vi "Connect CAN Adapter.vi"(8 "error in (no error)":errorcluster, 9 "Baud Rate":T1(ring), 10 "CAN Adapter Class Name":string, 11 "CANopen Master in":refnum<class "CANopen Master.lvclass">) -> (0 "error out":errorcluster, 3 "CANopen Master out":refnum<class "CANopen Master.lvclass">)   [LabVIEW 2024, in "CANopen Master.lvlib" / "CANopen Master.lvclass"]
uses:
  CANopen Master/CANopen Master.lvclass
  HAL/HAL/Configurations/CFG Base/CFG Base.lvclass
  HAL/HAL/Protocols/ICAN/ICAN.lvclass
  CANopen Master/CANopen Master.lvclass/CANopen Master.ctl
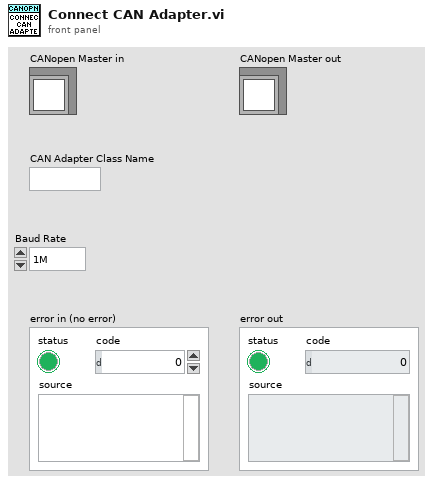
[diagram p1: front panel]
types:
  T1 = enum16{"1M", "800k", "500k", "250k", "125k", "50k", "25k", "10k"}
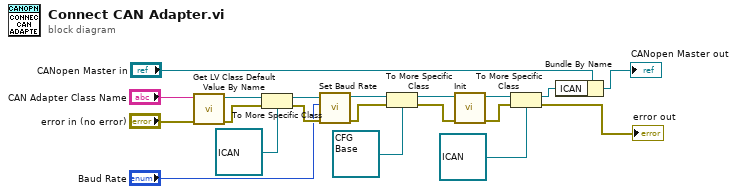
[diagram p0: block diagram]
diagram:
  n1 = call <vilib>:"Get LV Class Default Value By Name.vi"("error in (no error)"="error in (no error)", "class name"="CAN Adapter Class Name") -> ("error out"=w7:errorcluster, "object"=w16:refnum<class>)  [unwired: 8 in]
  n2 = To More Specific Class(target class=refnum<class "ICAN.lvclass"> refnum ("ICAN.lvclass"), reference=w16, error in=w7) -> (specific class reference=w8:refnum<class "ICAN.lvclass">, error out=w10:errorcluster)
  n3 = call-dynamic "Set Baud Rate.vi"("error in"=w10, "Baud Rate"="Baud Rate", "ICAN in"=w8) -> ("error out"=w14:errorcluster, "ICAN out"=w11:refnum<class "ICAN.lvclass">)  [unwired: 7 in]
  n4 = To More Specific Class(target class=refnum<class "CFG Base.lvclass"> refnum ("HAL.lvlib:CFG Base.lvclass"), reference=w11, error in=w14) -> (specific class reference=w13:refnum<class "CFG Base.lvclass">, error out=w15:errorcluster)
  n5 = call-dynamic "Init.vi"("error in"=w15, "CFG Base in"=w13) -> ("error out"=w12:errorcluster, "CFG Base out"=w19:refnum<class "CFG Base.lvclass">)  [unwired: 8 in]
  n6 = To More Specific Class(target class=refnum<class "ICAN.lvclass"> refnum ("ICAN.lvclass"), reference=w19, error in=w12) -> (specific class reference=w1:refnum<class "ICAN.lvclass">, error out=→"error out":errorcluster)
  n7 = Bundle By Name(cluster="CANopen Master in", "ICAN"=w1) -> (→"CANopen Master out":refnum<class "CANopen Master.lvclass">)
